vi "Calorimeter_2013.vi"() -> ()   [LabVIEW 2011]
uses:
  <vilib>/Instr/_visa.llb/VISA Flush IO Buffer Mask.ctl
  <vilib>/Utility/error.llb/DialogType.ctl
  <vilib>/Instr/_visa.llb/VISA Configure Serial Port (Instr).vi
  <vilib>/Utility/file.llb/Write To Spreadsheet File (DBL).vi
panel:
  in  "COM Port":refnum<visa-resource-name>="ASRL3::INSTR"
  in  "Temps":dbl[](array[numeric])
  out "Current Time":dbl
  in  "Times":dbl[](array[numeric])
  out "Temperature versus Time":cluster{dbl[], dbl[]}(graph)
  out "Temperature (C)":dbl format="%.3g"
  in  "Stop button":bool
  out "read buffer":string
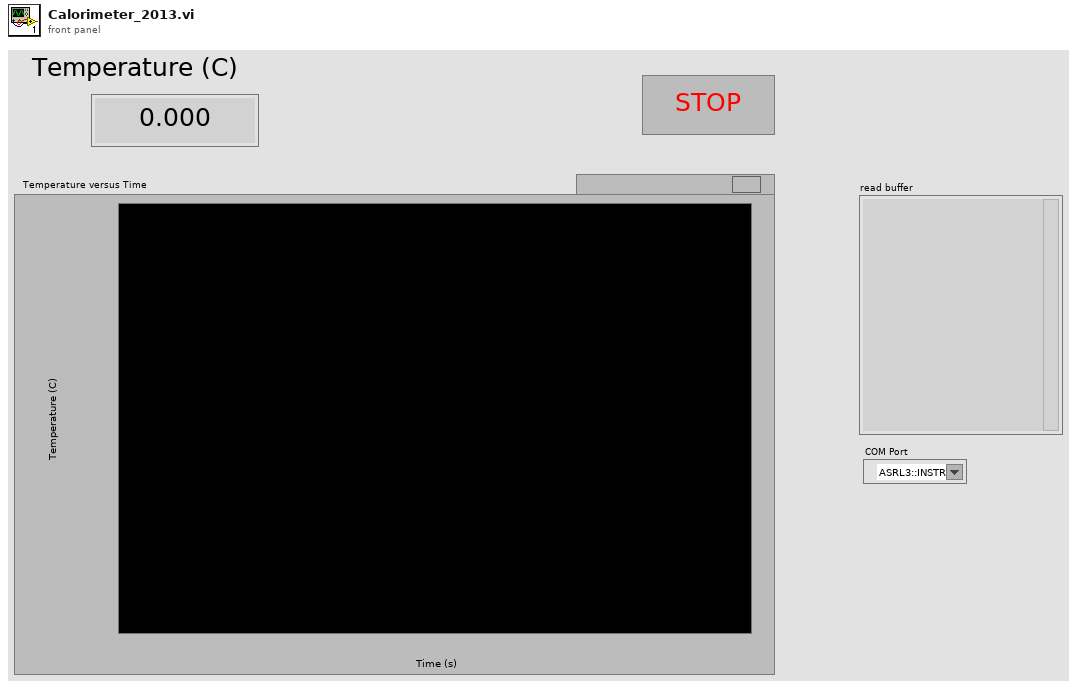
[diagram p1: front panel]
types:
  T1 = typedef "VISA Flush IO Buffer Mask.ctl" = u16
  T2 = typedef "DialogType.ctl" = u16
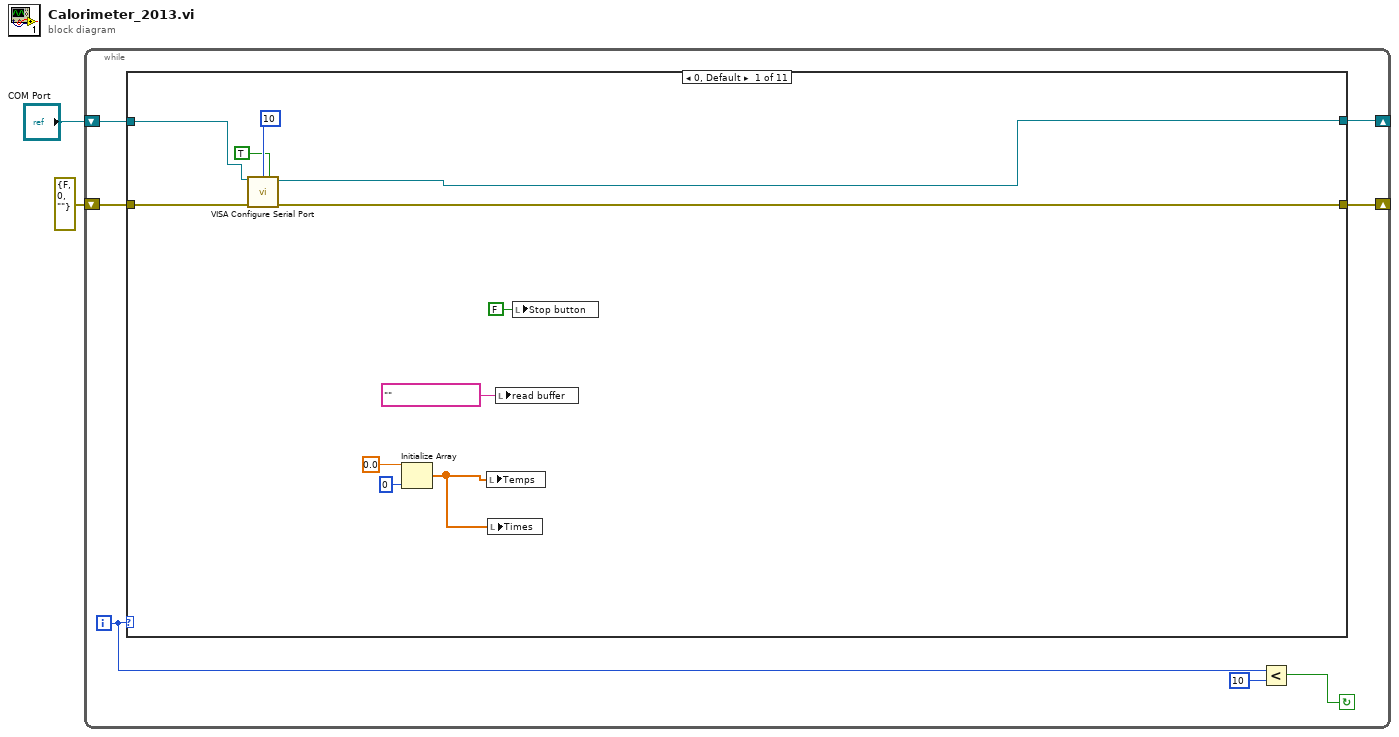
[diagram p0: block diagram]
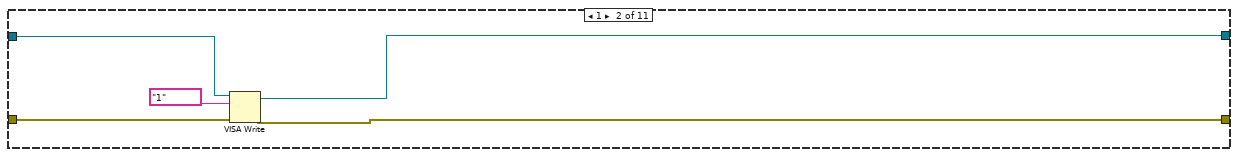
[diagram p2: hidden frame]
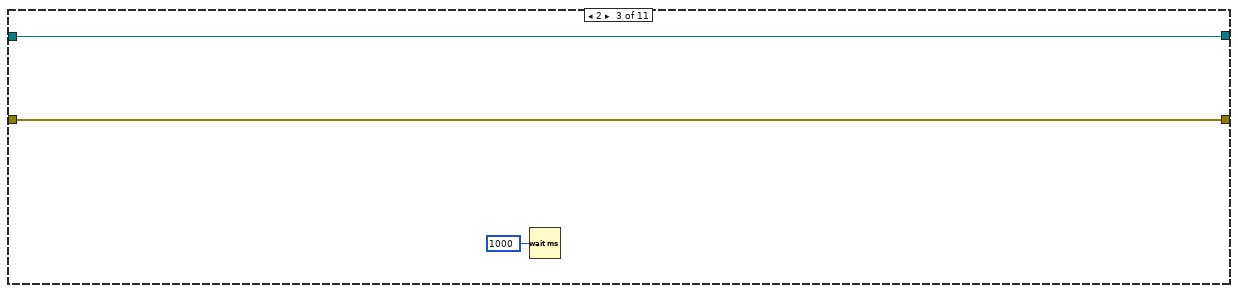
[diagram p3: hidden frame]
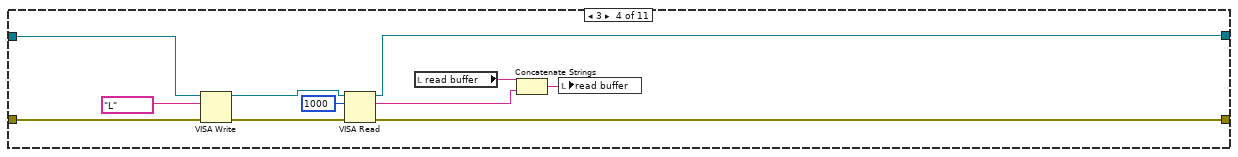
[diagram p4: hidden frame]
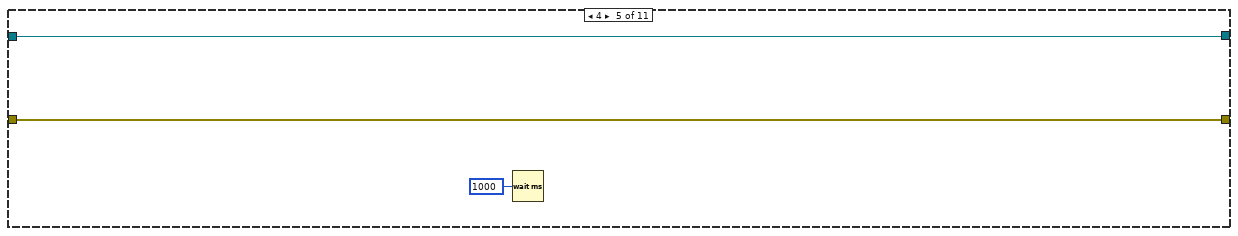
[diagram p5: hidden frame]
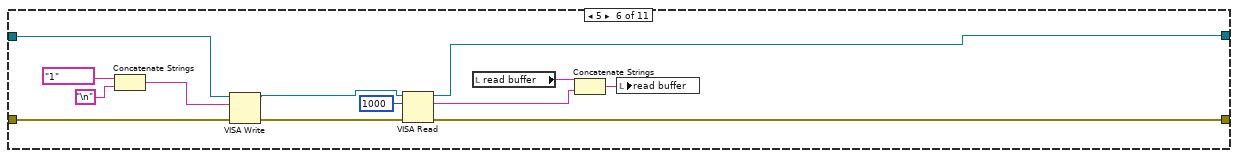
[diagram p6: hidden frame]
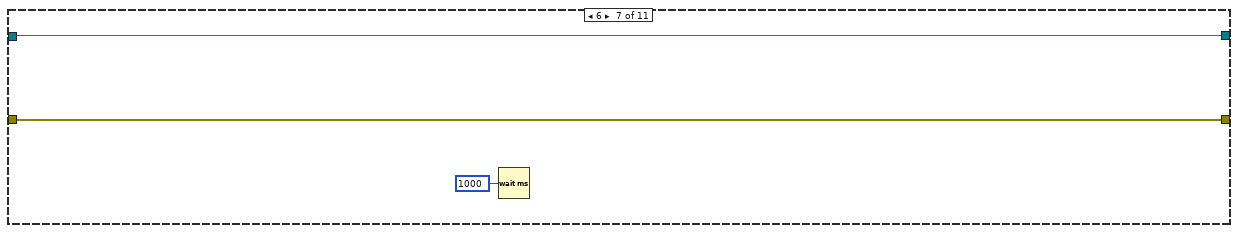
[diagram p7: hidden frame]
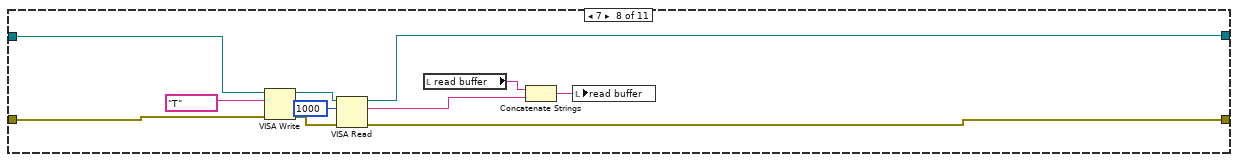
[diagram p8: hidden frame]
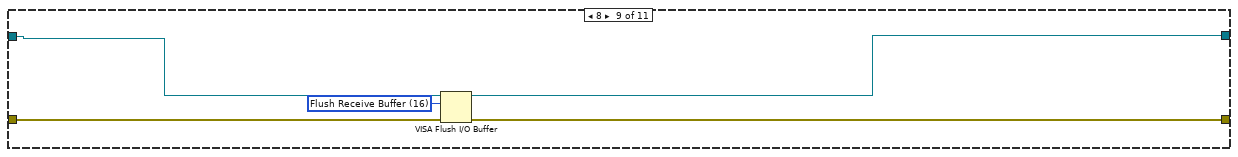
[diagram p9: hidden frame]
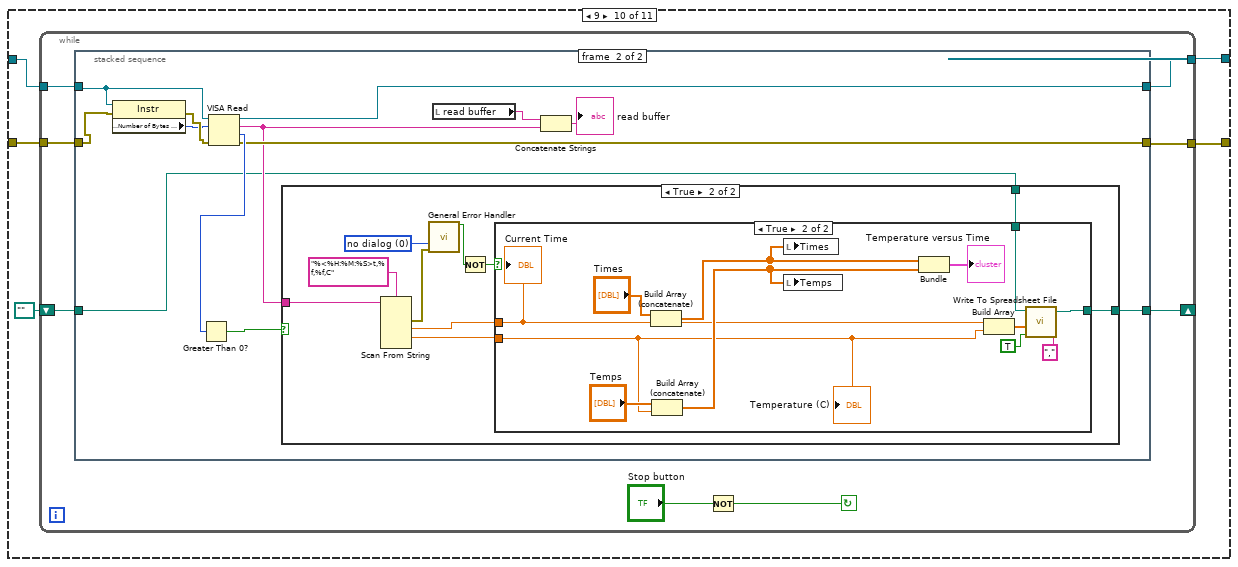
[diagram p10: hidden frame]
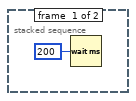
[diagram p11: hidden frame]
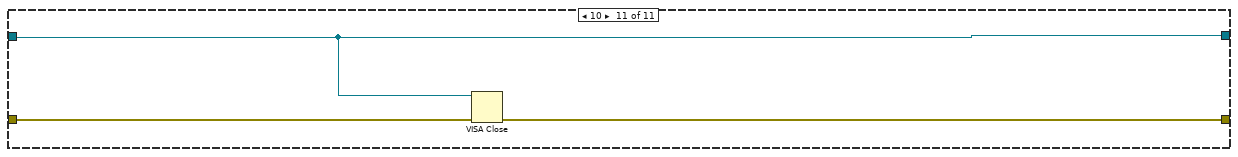
[diagram p14: hidden frame]
diagram:
  n1 = while {
    shift-right: [w5] -> _
    shift-left: "COM Port" -> [w9]
    shift-right: [w3] -> _
    shift-left: errorcluster {"status"=FALSE, "code"=0, "source"=""} ("error out") -> [w8]
    i -> [w7]
    stop <- w4 continue-if-true
    n2 = case shown="0, Default" w7 {
      tunnel: [w14 w21 w26 w29 w40 w43 w56 w60 w73 w79 w127] -> w3
      tunnel: w9 -> [w19 w24 w27 w38 w41 w55 w57 w67 w72 w77 w126]
      tunnel: [w15 w22 w27 w30 w41 w44 w57 w59 w70 w78 w126] -> w5
      tunnel: w8 -> [w20 w23 w26 w37 w40 w54 w56 w68 w74 w76 w128]
      frame 0, Default {
        n3 = call-poly "VISA Configure Serial Port"("VISA resource name"=w19, "termination char\n(0xA = '\\n' = LF)"=u8 10 ("termination char\n(0xA = '\\n' = LF)"), "Enable Termination\nChar (T)"=TRUE ("Enable Termination\nChar (T)"), "error in (no error)"=w20) -> ("VISA resource name out"=w15:refnum<visa-resource-name>, "error out"=w14:errorcluster)  [unwired: 10 in]
        n4 = Initialize Array(0.0 ("element"), 0 ("dimension size")) -> (w10:dbl[])
        n5 = local write "Temps"(w10) -> ()
        n6 = local write "Times"(w10) -> ()
        n7 = local write "read buffer"("" ("read buffer")) -> ()
        n8 = local write "Stop button"(FALSE ("Stop button")) -> ()
      }
      frame 1 {
        n9 = VISA Write(VISA resource name=w24, write buffer="1", error in (no error)=w23) -> (VISA resource name out=w22:refnum<visa-resource-name>, error out=w21:errorcluster)  [unwired: 1 out]
      }
      frame 2 {
        n10 = Wait (ms)(milliseconds to wait=u32 1000) -> ()  [unwired: 1 out]
      }
      frame 3 {
        n11 = VISA Write(VISA resource name=w38, write buffer="L", error in (no error)=w37) -> (VISA resource name out=w31:refnum<visa-resource-name>, error out=w32:errorcluster)  [unwired: 1 out]
        n12 = VISA Read(VISA resource name=w31, byte count=u32 1000, error in (no error)=w32) -> (VISA resource name out=w30:refnum<visa-resource-name>, read buffer=w33:string, error out=w29:errorcluster)  [unwired: 1 out]
        n13 = local read "read buffer"() -> (w34:string)
        n14 = Concatenate Strings(w34, w33) -> (w35:string)
        n15 = local write "read buffer"(w35) -> ()
      }
      frame 4 {
        n16 = Wait (ms)(milliseconds to wait=u32 1000) -> ()  [unwired: 1 out]
      }
      frame 5 {
        n17 = Concatenate Strings("1" ("write buffer"), "\n") -> (w51:string)
        n18 = VISA Write(VISA resource name=w55, write buffer=w51, error in (no error)=w54) -> (VISA resource name out=w45:refnum<visa-resource-name>, error out=w46:errorcluster)  [unwired: 1 out]
        n19 = VISA Read(VISA resource name=w45, byte count=u32 1000, error in (no error)=w46) -> (VISA resource name out=w44:refnum<visa-resource-name>, read buffer=w47:string, error out=w43:errorcluster)  [unwired: 1 out]
        n20 = local read "read buffer"() -> (w48:string)
        n21 = Concatenate Strings(w48, w47) -> (w49:string)
        n22 = local write "read buffer"(w49) -> ()
      }
      frame 6 {
        n23 = Wait (ms)(milliseconds to wait=u32 1000) -> ()  [unwired: 1 out]
      }
      frame 7 {
        n24 = VISA Write(VISA resource name=w67, write buffer="T", error in (no error)=w68) -> (VISA resource name out=w62:refnum<visa-resource-name>, error out=w61:errorcluster)  [unwired: 1 out]
        n25 = VISA Read(VISA resource name=w62, byte count=u32 1000, error in (no error)=w61) -> (VISA resource name out=w59:refnum<visa-resource-name>, read buffer=w64:string, error out=w60:errorcluster)  [unwired: 1 out]
        n26 = local read "read buffer"() -> (w65:string)
        n27 = Concatenate Strings(w65, w64) -> (w63:string)
        n28 = local write "read buffer"(w63) -> ()
      }
      frame 8 {
        w71 = T1 16 items=["Flush Receive Buffer"=16, "Write Transmit Buffer to Device"=32, "Flush Receive Buffer (No I/O)"=64, "Flush Transmit Buffer"=128] ("Mask")
        n29 = VISA Flush I/O Buffer(VISA resource name=w72, mask (16)=w71, error in (no error)=w74) -> (VISA resource name out=w70:refnum<visa-resource-name>, error out=w73:errorcluster)
      }
      frame 9 {
        n30 = while {
          tunnel: [w82] -> w79
          tunnel: [w84] -> w78
          tunnel: w77 -> [w87]
          tunnel: w76 -> [w86]
          shift-right: [w81] -> _
          shift-left: path "" ("new file path (Not A Path if cancelled)") -> [w80]
          stop <- w83 continue-if-true
          n31 = stacked-sequence {
            tunnel: w87 -> [_ w94]
            tunnel: w86 -> [_ w93]
            tunnel: [_ w101] -> w84
            tunnel: [_ w98] -> w82
            tunnel: [_ w90] -> w81
            tunnel: w80 -> [_ w89]
            frame #0 {
              n32 = Wait (ms)(milliseconds to wait=u32 200) -> ()  [unwired: 1 out]
            }
            frame #1 {
              n33 = property class="Instr"(reference=w94, error in=w93) -> (error out=w92:errorcluster, "Serial Settings:Number of Bytes at Serial Port"=w91:u32)  [unwired: 1 out]
              n34 = VISA Read(VISA resource name=w94, byte count=w91, error in (no error)=w92) -> (VISA resource name out=w101:refnum<visa-resource-name>, read buffer=w95:string, return count=w99:u32, error out=w98:errorcluster)
              n35 = Greater Than 0?(x=w99) -> (x > 0?=w100:bool)
              n36 = case shown="True" w100 {
                tunnel: w95 -> [_ w112]
                tunnel: [w102 w104] -> w90
                tunnel: w89 -> [w102 w103]
                frame False {
                }
                frame True {
                  w110 = T2 0 items=["no dialog", "OK message", "continue or stop message", "OK message + warnings", "continue/stop + warnings"] ("type of dialog (OK msg:1)")
                  n37 = Scan From String(format string="%<%H:%M:%S>t,%f,%f,C", input string=w112) -> (error out=w109:errorcluster, output 1=w105:dbl, output 2=w108:dbl)  [unwired: 6 in, 2 out]
                  n38 = call <vilib>:"General Error Handler.vi"("type of dialog (OK msg:1)"=w110, "error in (no error)"=w109) -> ("error?"=w107:bool)  [unwired: 9 in, 4 out]
                  n39 = Not(x=w107) -> (.not. x?=w106:bool)
                  n40 = case shown="True" w106 {
                    tunnel: w108 -> [_ w117]
                    tunnel: w105 -> [_ w118]
                    tunnel: [w113 w121] -> w104
                    tunnel: w103 -> [w113 w120]
                    frame False {
                    }
                    frame True {
                      n41 = Build Array (concatenate)("Times", w118) -> (w119:dbl[])
                      n42 = Build Array (concatenate)("Temps", w117) -> (w123:dbl[])
                      n43 = local write "Times"(w119) -> ()
                      n44 = local write "Temps"(w123) -> ()
                      n45 = Bundle(w119, w123) -> (→"Temperature versus Time":cluster{dbl[], dbl[]})  [unwired: 1 in]
                      n46 = Build Array(w118, w117) -> (w116:dbl[])
                      n47 = call-poly <vilib>:"Write To Spreadsheet File.vi"("delimiter (\\t)"="," ("delimiter (\\t)"), "append to file? (new file:F)"=TRUE, "1D data"=w116, "file path (dialog if empty)"=w120) -> ("new file path (Not A Path if cancelled)"=w121:path)  [unwired: 4 in]
                      "Temperature (C)" <- w117
                      "Current Time" <- w118
                    }
                  }
                }
              }
              n48 = local read "read buffer"() -> (w96:string)
              n49 = Concatenate Strings(w96, w95) -> (→"read buffer":string)
            }
          }
          n50 = Not(x="Stop button") -> (.not. x?=w83:bool)
        }
      }
      frame 10 {
        n51 = VISA Close(VISA resource name=w126, error in (no error)=w128) -> (error out=w127:errorcluster)
      }
    }
    n52 = Less?(x=w7, y=10) -> (x < y?=w4:bool)
  }
